vi "Configure.vi"(8 "error in (no error)":errorcluster, 11 "ConfocalStage in":refnum<class "ConfocalStage.lvclass">) -> (0 "error out":errorcluster, 2 "cancelled?":bool, 3 "ConfocalStage out":refnum<class "ConfocalStage.lvclass">)   [LabVIEW 2012, in "ConfocalStage.lvclass"]
doc: "The configure method configures the details for the RabbitMQ connection, the observers and the mapping script.\n\nIn the derived class, make a call to the parent for setting these parameters."
uses:
  ConfocalStage.lvclass
  <vilib>/Utility/miscctls.llb/LVPointTypeDef.ctl
  ConfocalStage.lvclass/ConfocalStage.ctl
  <vilib>/Distrio/Murmex/Murmex/Murmex.lvclass
panel:
  in  "button:cancel":bool
  in  "button:configure murmex":bool
  in  "button:ok":bool
  in  "Tab Control":enum32{"VISA", "Stages"}(tab)
  in  "stop bits":u16(ring)=20 items=["1.0"=10, "1.5"=15, "2.0"=20]
  in  "flow control":u16(ring) items=["None", "XON/XOFF", "RTS/CTS", "XON/XOFF & RTS/CTS", "DTR/DSR", "XON/XOFF & DTR/DSR"]
  in  "baud rate":u32
  in  "data bits":u16
  in  "send termination char?":bool
  in  "termination char":u8
  in  "parity (0:none)":enum16{"None", "Odd", "Even", "Mark", "Space"}(ring)
  in  "COM port":refnum<visa-resource-name>
  in  "position conversion focus":dbl
  in  "position conversion Y":dbl
  in  "position conversion X":dbl
  in  "speed conversion":dbl
  in  "accelleration ramp":dbl[unit]
  in  "startup speed":dbl[unit]
  # "(CarriageReturn=13)"
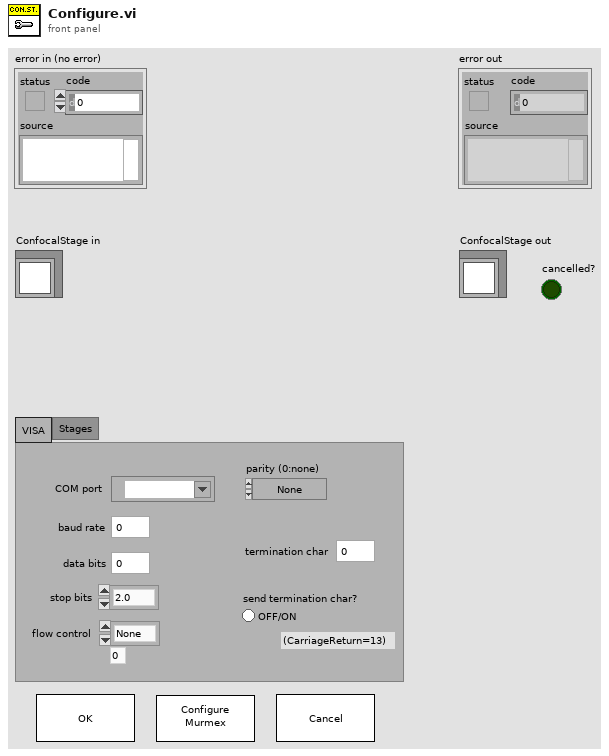
[diagram p1: front panel]
types:
  T1 = typedef "LVPointTypeDef.ctl" = cluster{"Horizontal":i16, "Vertical":i16}
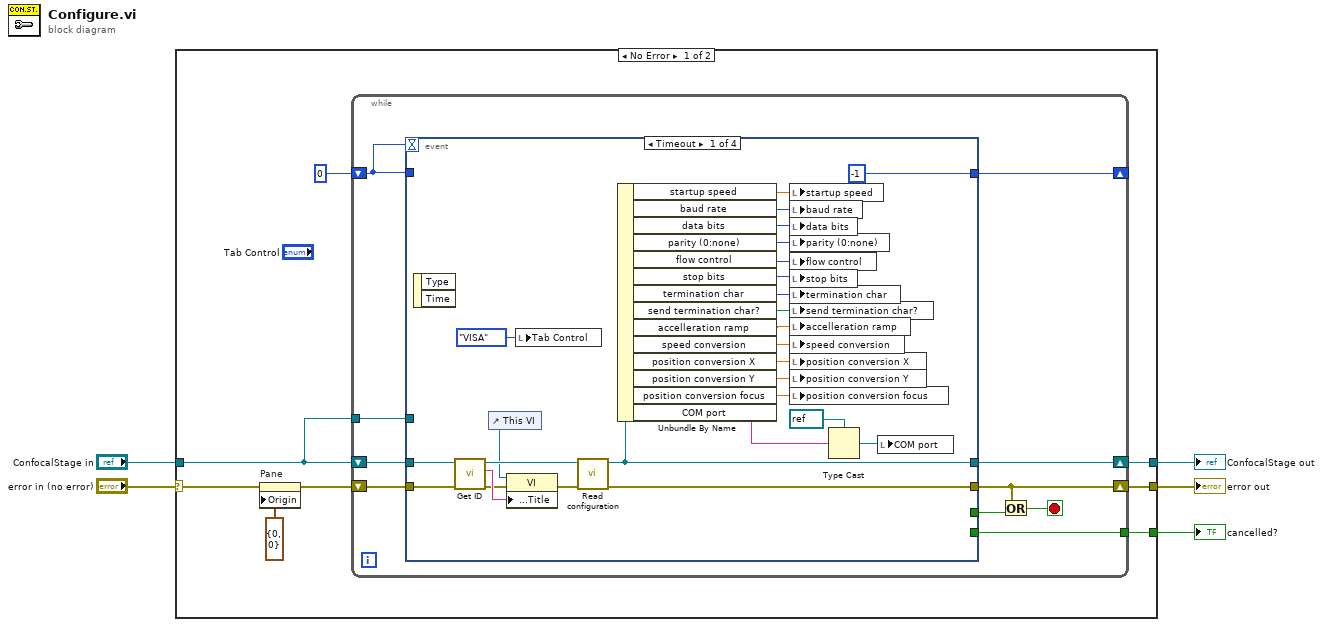
[diagram p0: block diagram]
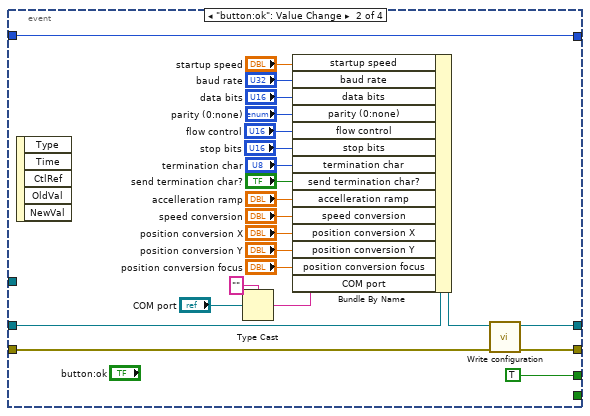
[diagram p2: hidden frame]
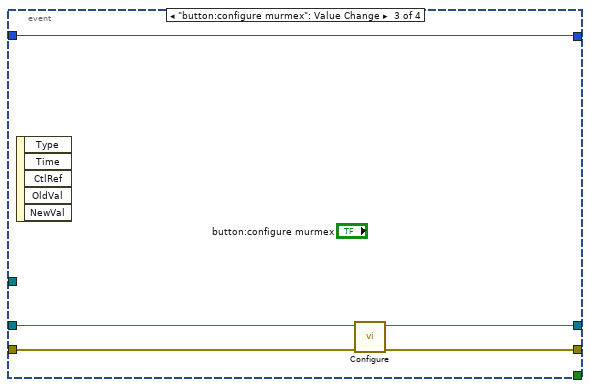
[diagram p3: hidden frame]
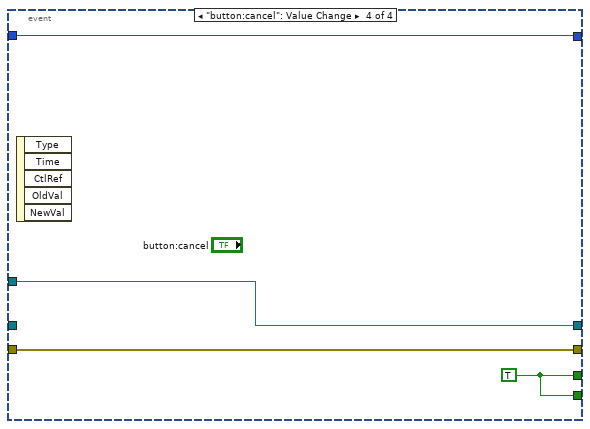
[diagram p4: hidden frame]
diagram:
  n1 = case shown="No Error" "error in (no error)" {
    selector: "error in (no error)" -> [w12 w83]
    tunnel: "ConfocalStage in" -> [w10 w84]
    tunnel: [w8 w83] -> w3
    tunnel: [w7 w84] -> w2
    tunnel: [w6 _] -> w1
    frame No Error {
      n2 = property on="Pane" class="Pane"(error in=w12, "Origin"=T1 {"Horizontal"=0, "Vertical"=0}) -> (error out=w11:errorcluster)  [unwired: 1 in, 1 out]
      n3 = while {
        shift-right: [w21] -> w7
        shift-left: w10 -> [w22]
        shift-right: [w18] -> w8
        shift-left: w11 -> [w23]
        tunnel: w10 -> [w15]
        shift-right: [w20] -> _
        shift-left: 0 -> [w19]
        tunnel: [w14] -> w6
        stop <- w16 stop-if-true
        n4 = event shown="[0] Timeout" {
          selector: _ -> [_ _ _ _]
          dyn-events: _ -> [_ _ _ _]
          timeout: w19 -> [_ _ _ _]
          tunnel: w23 -> [w44 w72 w78 w80]
          tunnel: w22 -> [w43 w69 w77 _]
          tunnel: [w29 w70 w76 w81] -> w21
          tunnel: [-1 w73 w74 w82] -> w20
          tunnel: w19 -> [_ w73 w74 w82]
          tunnel: [w27 w71 w75 w80] -> w18
          tunnel: [_ TRUE _ w79] -> w17
          tunnel: w15 -> [_ _ _ w81]
          tunnel: [_ _ _ w79] -> w14
          event Timeout {
            n5 = event-data() -> ()  [unwired: 1 in, 2 out]
            n6 = call <vilib>:"Get ID.vi"("error in (no error)"=w44, "Murmex in"=w43) -> ("error out"=w45:errorcluster, "component id"=w49:string, "Murmex out"=w48:refnum<class "ConfocalStage.lvclass">)  [unwired: 7 in]
            n7 = control-ref of="This VI"() -> (w46:refnum<vi>)
            n8 = property class="VI"(reference=w46, error in=w45, "Front Panel.Title"=w49) -> (error out=w47:errorcluster)  [unwired: 1 out]
            n9 = local write "Tab Control"(enum32{"VISA", "Stages"}."VISA" ("Tab Control")) -> ()
            n10 = call <vilib>:"Read configuration.vi"("error in (no error)"=w47, "Murmex in"=w48) -> ("error out"=w27:errorcluster, "Murmex out"=w29:refnum<class "ConfocalStage.lvclass">)  [unwired: 7 in, 1 out]
            n11 = Unbundle By Name(w29) -> ("startup speed"=w42:dbl[unit], "baud rate"=w41:u32, "data bits"=w31:u16, "parity (0:none)"=w38:enum16{"None", "Odd", "Even", "Mark", "Space"}, "flow control"=w37:u16, "stop bits"=w40:u16, "termination char"=w39:u8, "send termination char?"=w30:bool, "accelleration ramp"=w32:dbl[unit], "speed conversion"=w35:dbl, "position conversion X"=w33:dbl, "position conversion Y"=w34:dbl, "position conversion focus"=w36:dbl, "COM port"=w26:string)
            n12 = local write "startup speed"(w42) -> ()
            n13 = local write "baud rate"(w41) -> ()
            n14 = local write "data bits"(w31) -> ()
            n15 = local write "parity (0:none)"(w38) -> ()
            n16 = local write "flow control"(w37) -> ()
            n17 = local write "stop bits"(w40) -> ()
            n18 = local write "termination char"(w39) -> ()
            n19 = local write "send termination char?"(w30) -> ()
            n20 = local write "accelleration ramp"(w32) -> ()
            n21 = local write "speed conversion"(w35) -> ()
            n22 = local write "position conversion X"(w33) -> ()
            n23 = local write "position conversion Y"(w34) -> ()
            n24 = local write "position conversion focus"(w36) -> ()
            n25 = Type Cast(type=refnum<visa-resource-name> refnum ("COM port"), x=w26) -> (*(type *) &x=w24:refnum<visa-resource-name>)
            n26 = local write "COM port"(w24) -> ()
          }
          event "button:ok": Value Change {
            n27 = event-data() -> ()  [unwired: 1 in, 5 out]
            n28 = Type Cast(type="" ("configuration.Serial port.COM port"), x="COM port") -> (*(type *) &x=w52:string)
            n29 = Bundle By Name(cluster=w69, "startup speed"="startup speed", "baud rate"="baud rate", "data bits"="data bits", "parity (0:none)"="parity (0:none)", "flow control"="flow control", "stop bits"="stop bits", "termination char"="termination char", "send termination char?"="send termination char?", "accelleration ramp"="accelleration ramp", "speed conversion"="speed conversion", "position conversion X"="position conversion X", "position conversion Y"="position conversion Y", "position conversion focus"="position conversion focus", "COM port"=w52) -> (w68:refnum<class "ConfocalStage.lvclass">)
            n30 = call <vilib>:"Write configuration.vi"("error in (no error)"=w72, "Murmex in"=w68) -> ("error out"=w71:errorcluster, "Murmex out"=w70:refnum<class "ConfocalStage.lvclass">)  [unwired: 8 in]
          }
          event "button:configure murmex": Value Change {
            n31 = event-data() -> ()  [unwired: 1 in, 5 out]
            n32 = call-parent "Configure.vi"("error in (no error)"=w78, "Murmex in"=w77) -> ("error out"=w75:errorcluster, "Murmex out"=w76:refnum<class "ConfocalStage.lvclass">)  [unwired: 7 in, 1 out]
          }
          event "button:cancel": Value Change {
            w79 = TRUE
            n33 = event-data() -> ()  [unwired: 1 in, 5 out]
          }
        }
        n34 = Or(x=w18, y=w17) -> (x .or. y?=w16:bool)
      }
    }
    frame Error {
    }
  }
  "error out" <- w3
  "ConfocalStage out" <- w2
  "cancelled?" <- w1
